vi "Ch DecToHex Str.vi"(3 "Channel To Modify":u16 max=10) -> (0 "Array HexDec":u8[](array[numeric]), 1 "Str Hex Dec":string)   [LabVIEW 2018]
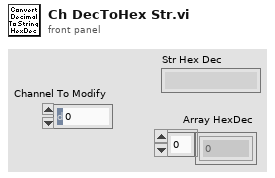
[diagram p1: front panel]
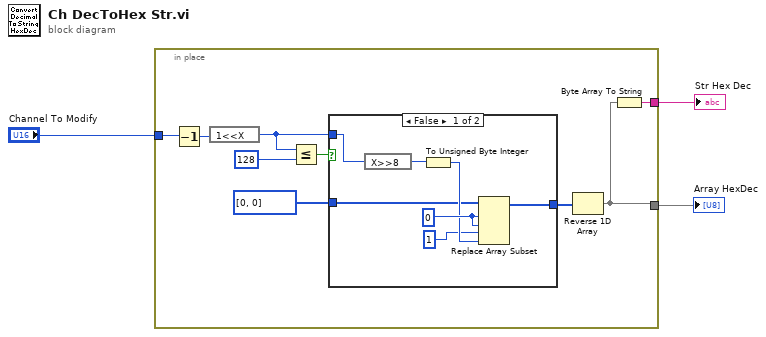
[diagram p0: block diagram]
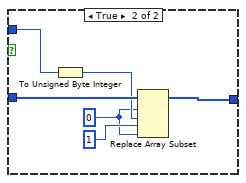
[diagram p2: hidden frame]
diagram:
  n1 = in-place {
    in-place-border: "Channel To Modify" -> [w12]
    in-place-border: [w7] -> w2
    in-place-border: [w4] -> w1
    n2 = Decrement(x=w12) -> (x-1=w11:u16)
    n3 = expression code="1<<X"(w11) -> (w8:u16)
    n4 = Less Or Equal?(x=w8, y=u16 128) -> (x <= y?=w10:bool)
    n5 = case shown="False" w10 {
      tunnel: u8[] [0, 0] -> [w13 w25]
      tunnel: [w19 w24] -> w5
      tunnel: w8 -> [w17 w22]
      frame False {
        w16 = 0 ("index")
        n6 = expression code="X>>8"(w17) -> (w18:u16)
        n7 = To Unsigned Byte Integer(number=w18) -> (unsigned 8bit integer=w15:u8)
        n8 = Replace Array Subset(array=w13, new element #1=w16, index #1=w16, new element #2=w15, index #2=1 ("index")) -> (w19:u8[])
      }
      frame True {
        w20 = 0 ("index")
        n9 = To Unsigned Byte Integer(number=w22) -> (unsigned 8bit integer=w21:u8)
        n10 = Replace Array Subset(array=w25, new element #1=w21, index #1=w20, new element #2=w20, index #2=1 ("index")) -> (w24:u8[])
      }
    }
    n11 = Reverse 1D Array(array=w5) -> (reversed array=w4:u8[])
    n12 = Byte Array To String(unsigned byte array=w4) -> (string=w7:string)
  }
  "Str Hex Dec" <- w2
  "Array HexDec" <- w1
